vi "Add Panel Intro.vi"(10 "connection information":path, 11 "System Number":dbl=1.0 format="%#_13g") -> ()   [LabVIEW 2024]
uses:
  <vilib>/addons/database/Connection.llb/DB Tools Open Connec (Path).vi
  <vilib>/addons/database/Connection.llb/DB Tools Open Connec (String).vi
  <vilib>/addons/database/_DB Variant To Data/Database Variant To Data.xnode
  <vilib>/regexp/Match Regular Expression.xnode
  <vilib>/addons/database/NI_Database_API.lvlib
panel:
  in  "PartNumber":string
  in  "Voltage":string
  in  "Waveform":string
  in  "Work Order":string
  in  "Bottom Rack Serial Number":string
  in  "Frequency (MHz)":string
  in  "User":string
  in  "Work Order (Subnumber)":string
  in  "Top Rack Serial Number":string
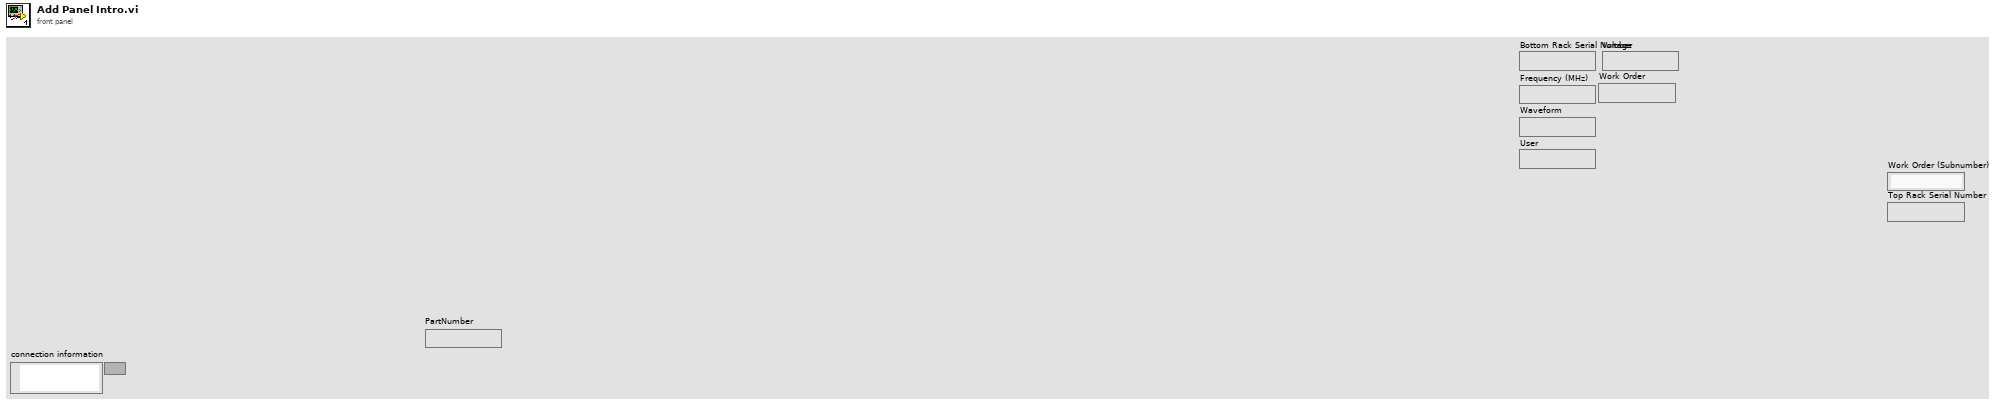
[diagram p1: front panel]
types:
  T1 = typedef "NI_Database_API.lvlib/Conn ObjectReference.ctl" = refnum<k1>
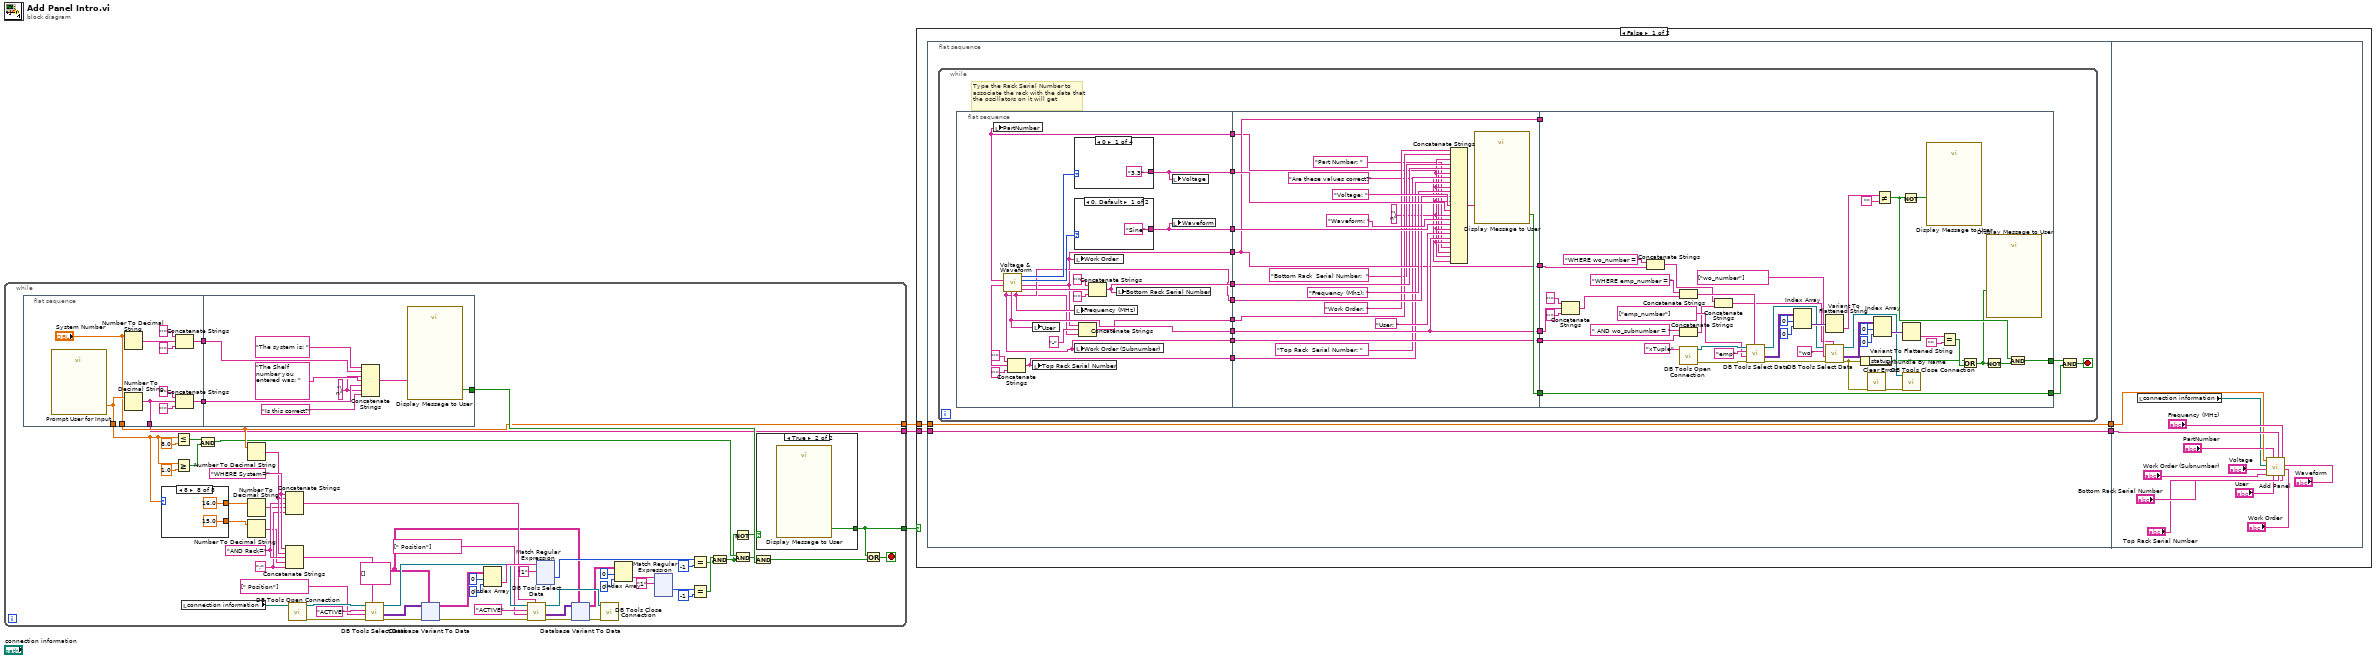
[diagram p0: block diagram]
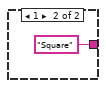
[diagram p2: hidden frame]
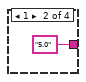
[diagram p3: hidden frame]
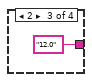
[diagram p4: hidden frame]
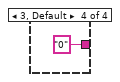
[diagram p5: hidden frame]
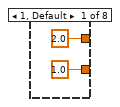
[diagram p7: hidden frame]
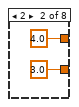
[diagram p8: hidden frame]
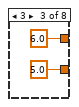
[diagram p9: hidden frame]
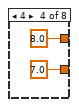
[diagram p10: hidden frame]
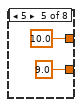
[diagram p11: hidden frame]
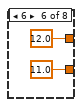
[diagram p12: hidden frame]
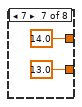
[diagram p13: hidden frame]
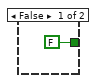
[diagram p14: hidden frame]
diagram:
  n1 = while {
    tunnel: [w55] -> w2
    tunnel: [w26] -> w1
    tunnel: [w43] -> w3
    stop <- w45 stop-if-true
    w7 = string[][] [] ("table")
    w40 = "AND Rack=" ("string")
    w39 = ";" ("string")
    w42 = "WHERE System=" ("SQL Query")
    n2 = flat-sequence {
      tunnel: [w403] -> w58
      tunnel: [w410] -> w38
      tunnel: ["System Number"] -> w55
      tunnel: [w406] -> w56
      tunnel: [w404] -> w26
      tunnel: w58 -> [w420]
      tunnel: [w416] -> w57
      tunnel: w56 -> [w413]
      frame #0 {
        n3 = call "Prompt User for Input"() -> ("Shelf Number"=w410:dbl)  [unwired: 17 in, 2 out]
        n4 = Number To Decimal String(number="System Number") -> (decimal integer string=w407:string)  [unwired: 1 in]
        n5 = Number To Decimal String(number=w410) -> (decimal integer string=w404:string)  [unwired: 1 in]
        n6 = Concatenate Strings("'" ("string"), w407, "'" ("string")) -> (w406:string)
        n7 = Concatenate Strings("'" ("string"), w404, "'" ("string")) -> (w403:string)
      }
      frame #1 {
        w414 = "\n" ("string")
        n8 = Concatenate Strings("The system is: " ("string"), w413, w414, "The Shelf number you entered was: " ("string"), w420, w414, "Is this correct?" ("string")) -> (w417:string)
        n9 = call "Display Message to User"("Message"=w417) -> ("Yes"=w416:bool)  [unwired: 9 in, 1 out]
      }
    }
    n10 = case shown="8" w38 {
      tunnel: [1.0 ("y") 3.0 ("y") 5.0 ("y") 7.0 ("y") 9.0 ("y") 11.0 ("y") 13.0 ("y") 15.0 ("y")] -> w36
      tunnel: [2.0 ("y") 4.0 ("y") 6.0 ("y") 8.0 ("y") 10.0 ("y") 12.0 ("y") 14.0 ("y") 16.0 ("y")] -> w37
      frame 1, Default {
      }
      frame 2 {
      }
      frame 3 {
      }
      frame 4 {
      }
      frame 5 {
      }
      frame 6 {
      }
      frame 7 {
      }
      frame 8 {
      }
    }
    n11 = Less Or Equal?(x=w38, y=8.0) -> (x <= y?=w61:bool)
    n12 = Greater Or Equal?(x=w38, y=1.0) -> (x >= y?=w62:bool)
    n13 = local read "connection information"() -> (w6:path)
    n14 = And(x=w61, y=w62) -> (x .and. y?=w48:bool)
    n15 = Number To Decimal String(number=w55) -> (decimal integer string=w41:string)  [unwired: 1 in]
    n16 = Number To Decimal String(number=w37) -> (decimal integer string=w25:string)  [unwired: 1 in]
    n17 = Number To Decimal String(number=w36) -> (decimal integer string=w24:string)  [unwired: 1 in]
    n18 = Concatenate Strings(w42, w41, w40, w25, w39) -> (w16:string)
    n19 = Concatenate Strings(w42, w41, w40, w24, w39) -> (w15:string)
    n20 = call-poly <vilib>:"DB Tools Open Connection.vi"("connection information"=w6) -> ("error out"=w22:errorcluster, "connection reference"=w23:T1)  [unwired: 7 in]
    n21 = call <vilib>:"DB Tools Select Data.vi"("condition"=w15, "error in (no error)"=w22, "columns"=string[] [" Position"], "table"="ACTIVE", "connection reference"=w23) -> ("error out"=w13:errorcluster, "data"=w20:variant[][], "connection reference out"=w18:T1)  [unwired: 1 in]
    n22 = xnode "Database Variant To Data"("database variant"=w20, "error in (no error)"=w13, "type"=w7) -> ("data"=w14:string[][], "error out"=w12:errorcluster)
    n23 = Index Array(array=w14, index (row)=0, index (col)=0 ("disabled index (col)")) -> (element=w52:string)
    n24 = call <vilib>:"DB Tools Select Data.vi"("condition"=w16, "error in (no error)"=w12, "columns"=string[] [" Position"], "table"="ACTIVE", "connection reference"=w18) -> ("error out"=w11:errorcluster, "data"=w9:variant[][], "connection reference out"=w19:T1)  [unwired: 1 in]
    n25 = xnode "Match Regular Expression"("input string"=w52, "regular expression"="1") -> ("offset past match"=w50:i32)  [unwired: 4 in, 4 out]
    n26 = xnode "Database Variant To Data"("database variant"=w9, "error in (no error)"=w11, "type"=w7) -> ("data"=w8:string[][], "error out"=w10:errorcluster)
    n27 = call <vilib>:"DB Tools Close Connection.vi"("error in (no error)"=w10, "connection reference"=w19) -> ()  [unwired: 5 in, 1 out]
    n28 = Index Array(array=w8, index (row)=0, index (col)=0 ("disabled index (col)")) -> (element=w33:string)
    n29 = xnode "Match Regular Expression"("input string"=w33, "regular expression"="1") -> ("offset past match"=w31:i32)  [unwired: 4 in, 4 out]
    n30 = Equal?(x=w50, y=-1) -> (x = y?=w28:bool)
    n31 = Equal?(x=w31, y=-1) -> (x = y?=w29:bool)
    n32 = And(x=w29, y=w28) -> (x .and. y?=w27:bool)
    n33 = Not(x=w27) -> (.not. x?=w44:bool)
    n34 = And(x=w48, y=w27) -> (x .and. y?=w47:bool)
    n35 = And(x=w47, y=w57) -> (x .and. y?=w46:bool)
    n36 = case shown="True" w44 {
      tunnel: [FALSE w285] -> w43
      frame False {
      }
      frame True {
        n37 = call "Display Message to User"() -> ("Stop"=w285:bool)  [unwired: 10 in, 1 out]
      }
    }
    n38 = Or(x=w43, y=w46) -> (x .or. y?=w45:bool)
  }
  n39 = case shown="False" w3 {
    tunnel: w1 -> [w422 _]
    tunnel: w2 -> [w421 _]
    frame False {
      n40 = flat-sequence {
        tunnel: [w426] -> w424
        tunnel: [w425] -> w423
        tunnel: w422 -> [w426]
        tunnel: w421 -> [w425]
        tunnel: w424 -> [w548]
        tunnel: w423 -> [w541]
        frame #0 {
          n41 = while {
            stop <- w434 stop-if-true
            # "Type the Rack Serial Number to associate the rack with the data that the oscillators on it will get"
            n42 = flat-sequence {
              tunnel: [w461] -> w444
              tunnel: [w455] -> w443
              tunnel: [w454] -> w442
              tunnel: [w457] -> w441
              tunnel: [w452] -> w440
              tunnel: [w456] -> w439
              tunnel: [w451] -> w431
              tunnel: [w450] -> w429
              tunnel: [w446] -> w428
              tunnel: [w445] -> w427
              tunnel: w444 -> [w479]
              tunnel: w443 -> [w488]
              tunnel: w442 -> [w487]
              tunnel: w441 -> [w484]
              tunnel: w440 -> [w481]
              tunnel: w439 -> [w482]
              tunnel: [w490] -> w438
              tunnel: [w482] -> w437
              tunnel: [w481] -> w433
              tunnel: [w481] -> w432
              tunnel: w431 -> [w478]
              tunnel: [w480] -> w430
              tunnel: w429 -> [w480]
              tunnel: w428 -> [w476]
              tunnel: w427 -> [w470]
              tunnel: [w498] -> w436
              tunnel: [w536] -> w435
              tunnel: w430 -> [w513]
              tunnel: w432 -> [w517]
              tunnel: w433 -> [_]
              tunnel: w437 -> [w519]
              tunnel: w438 -> [w536]
              frame #0 {
                n43 = call "Voltage & Waveform.vi"() -> ("Bottom Rack Serial Number"=w458:string, "Work Order"=w452:string, "Waveform"=w459:u16, "Voltage"=w460:u16, "Frequency (MHz)"=w457:string, "User"=w456:string, "Work Order (Subnumber)"=w450:string, "Top Rack Serial Number"=w447:string, "PartNumber"=w445:string)  [unwired: 3 in]
                n44 = local write "PartNumber"(w445) -> ()
                n45 = Concatenate Strings("'" ("string"), w447, "'" ("string")) -> (w446:string)
                n46 = local write "User"(w456) -> ()
                n47 = local write "Top Rack Serial Number"(w446) -> ()
                n48 = case shown="0" w460 {
                  tunnel: ["3.3" "5.0" "12.0" "0"] -> w455
                  frame 0 {
                  }
                  frame 1 {
                  }
                  frame 2 {
                  }
                  frame 3, Default {
                  }
                }
                n49 = case shown="0, Default" w459 {
                  tunnel: ["Sine" "Square"] -> w454
                  frame 0, Default {
                  }
                  frame 1 {
                  }
                }
                n50 = local write "Work Order"(w452) -> ()
                n51 = local write "Frequency (MHz)"(w457) -> ()
                n52 = local write "Work Order (Subnumber)"(w450) -> ()
                n53 = Concatenate Strings(w452, "-" ("string"), w450) -> (w451:string)
                n54 = Concatenate Strings("'" ("string"), w458, "'" ("string")) -> (w461:string)
                n55 = local write "Bottom Rack Serial Number"(w461) -> ()
                n56 = local write "Voltage"(w455) -> ()
                n57 = local write "Waveform"(w454) -> ()
              }
              frame #1 {
                w472 = "\n" ("string")
                n58 = Concatenate Strings("Work Order: " ("string"), w478, w472, "Bottom Rack  Serial Number:  " ("string"), w479, w472, "Top Rack  Serial Number: " ("string"), w476, w472, "Frequency (Mhz): " ("string"), w484, w472, "Voltage: " ("string"), w488, w472, "Waveform: " ("string"), w487, w472, "User: " ("string"), w482, w472, "Part Number: " ("string"), w470, w472, "Are these values correct?" ("string")) -> (w491:string)
                n59 = call "Display Message to User"("Message"=w491) -> ("Yes"=w490:bool)  [unwired: 9 in, 1 out]
              }
              frame #2 {
                n60 = Concatenate Strings("'" ("string"), w519, "'" ("string")) -> (w518:string)
                n61 = Concatenate Strings("WHERE wo_number = " ("string"), w517) -> (w502:string)
                n62 = Concatenate Strings("WHERE emp_number = " ("condition"), w518) -> (w530:string)
                n63 = Concatenate Strings(" AND wo_subnumber = " ("string"), w513) -> (w501:string)
                n64 = call-poly <vilib>:"DB Tools Open Connection.vi"("connection information"="xTuple" ("Connection Strings")) -> ("error out"=w535:errorcluster, "connection reference"=w532:T1)  [unwired: 7 in]
                n65 = Concatenate Strings(w502, w501) -> (w500:string)
                n66 = call <vilib>:"DB Tools Select Data.vi"("condition"=w530, "error in (no error)"=w535, "columns"=string[] ["emp_number"], "table"="emp", "connection reference"=w532) -> ("error out"=w512:errorcluster, "data"=w526:variant[][], "connection reference out"=w509:T1)  [unwired: 1 in]
                n67 = Index Array(array=w526, index (row)=0, index (col)=0 ("disabled index (col)")) -> (element=w527:variant)
                n68 = Variant To Flattened String(Variant=w527) -> (data string=w524:string)  [unwired: 1 out]
                n69 = call <vilib>:"DB Tools Select Data.vi"("condition"=w500, "error in (no error)"=w512, "columns"=string[] ["wo_number"], "table"="wo", "connection reference"=w509) -> ("error out"=w497:errorcluster, "data"=w505:variant[][], "connection reference out"=w499:T1)  [unwired: 1 in]
                n70 = Unbundle By Name(w497) -> ("status"=w494:bool)
                n71 = call <vilib>:"Clear Errors.vi"("error in (no error)"=w497) -> ("error out"=w496:errorcluster)  [unwired: 5 in, 1 out]
                n72 = Index Array(array=w505, index (row)=0, index (col)=0 ("disabled index (col)")) -> (element=w504:variant)
                n73 = Not Equal?(x=w524, y="") -> (x != y?=w515:bool)
                n74 = Not(x=w515) -> (.not. x?=w523:bool)
                n75 = Variant To Flattened String(Variant=w504) -> (data string=w503:string)  [unwired: 1 out]
                n76 = call <vilib>:"DB Tools Close Connection.vi"("error in (no error)"=w496, "connection reference"=w499) -> ()  [unwired: 5 in, 1 out]
                n77 = call "Display Message to User"("Enable"=w523) -> ()  [unwired: 9 in, 2 out]
                n78 = Equal?(x=w503, y="") -> (x = y?=w495:bool)
                n79 = Or(x=w494, y=w495) -> (x .or. y?=w492:bool)
                n80 = Not(x=w492) -> (.not. x?=w493:bool)
                n81 = call "Display Message to User"("Enable"=w492) -> ()  [unwired: 9 in, 2 out]
                n82 = And(x=w515, y=w493) -> (x .and. y?=w498:bool)
              }
            }
            n83 = And(x=w436, y=w435) -> (x .and. y?=w434:bool)
          }
        }
        frame #1 {
          n84 = local read "connection information"() -> (w537:path)
          n85 = call "Add Panel.vi"("Top Rack Serial Number"="Top Rack Serial Number", "Work Order"="Work Order", "Waveform"="Waveform", "Frequency (MHz)"="Frequency (MHz)", "Bottom Rack Serial Number"="Bottom Rack Serial Number", "Shelf Number"=w548, "User"="User", "PartNumber"="PartNumber", "SubNumber"="Work Order (Subnumber)", "Voltage"="Voltage", "connection information"=w537, "System Num"=w541) -> ()
        }
      }
    }
    frame True {
    }
  }
